vi "Totalize.vi"(6 "gain":dbl=1.0 format="%_6g", 7 "timebase":T1 items=["Seconds", "Minutes", "Hours", "Days"], 8 "error in":errorcluster, 9 "reset":bool, 10 "input":dbl format="%_6g", 11 "enable":bool=TRUE) -> (0 "error out":errorcluster, 3 "total":dbl format="%_6g")   [LabVIEW 2017, in "NI_FunctionBlock Libraries.lvlib"]
uses:
  <vilib>/functionblocks/NI_FunctionBlock Libraries.lvlib
  <vilib>/functionblocks/Accumulate/Totalize/Totalize.ctl
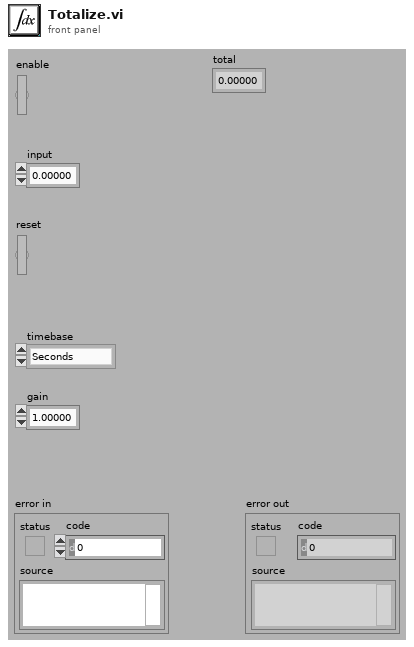
[diagram p1: front panel]
types:
  T1 = typedef "NI_FunctionBlock Libraries.lvlib/Totalize.ctl" = u16
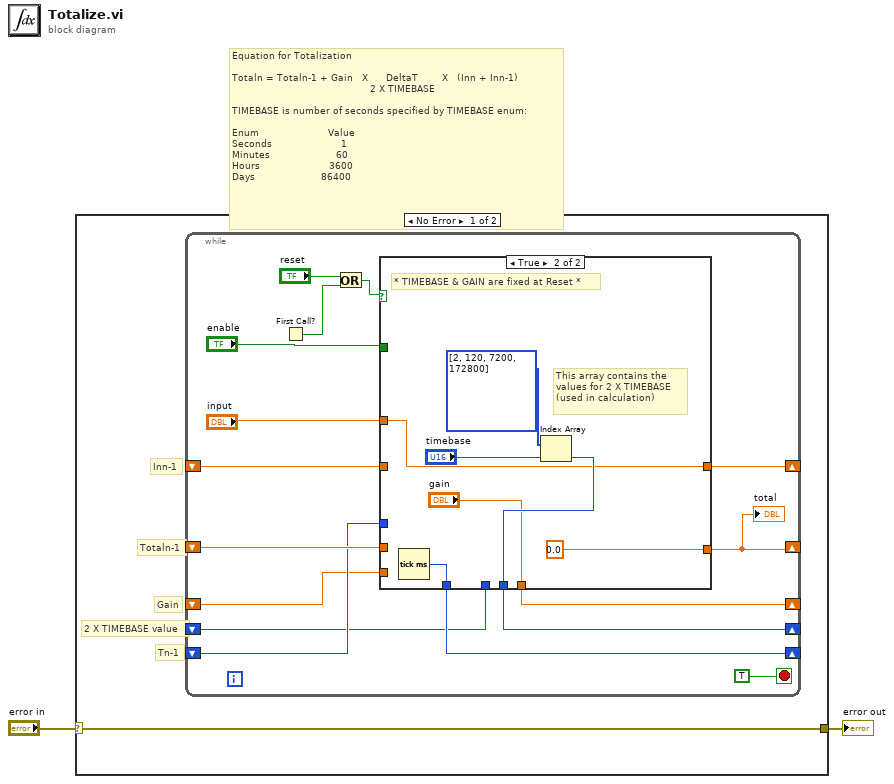
[diagram p0: block diagram]
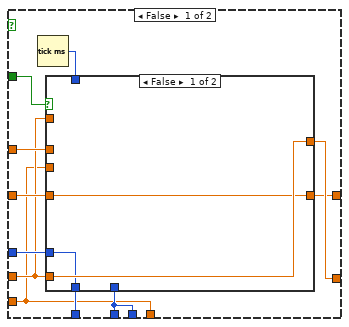
[diagram p2: hidden frame]
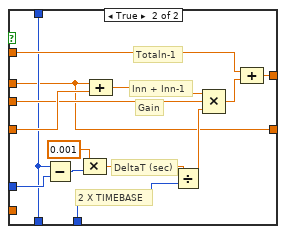
[diagram p3: hidden frame]
diagram:
  # "Equation for Totalization\n\nTotaln = Totaln-1 + Gain   X      DeltaT        X   (Inn + Inn-1)\n                                              2 X TIMEBASE\n\nTIMEBASE is number of seconds specified by TIMEBASE enum:\n\nEnum                       Value\nSeconds                       1\nMinutes                      60\nHours                       3600\nDays                      86400"
  n1 = case shown="No Error" "error in" {
    selector: "error in" -> [w3 w55]
    tunnel: [w3 w55] -> w1
    frame No Error {
      # "Gain"
      # "Tn-1"
      # "2 X TIMEBASE value"
      # "Totaln-1"
      # "Inn-1"
      n2 = while {
        shift-right: [w15] -> _
        shift-left: _ -> [w14]
        shift-right: [w4] -> _
        shift-left: _ -> [w13]
        shift-right: [w11] -> _
        shift-left: _ -> [w9]
        shift-right: [w10] -> _
        shift-left: _ -> [w12]
        shift-right: [w8] -> _
        shift-left: _ -> [w7]
        stop <- TRUE stop-if-true
        n3 = First Call?() -> (First Call?: T/F=w18:bool)
        n4 = Or(x="reset", y=w18) -> (x .or. y?=w17:bool)
        n5 = case shown="True" w17 {
          tunnel: [w28 0.0 ("Accumulation")] -> w15
          tunnel: "enable" -> [w30 _]
          tunnel: "input" -> [w29 w48]
          tunnel: w14 -> [w24 _]
          tunnel: w13 -> [w27 _]
          tunnel: w12 -> [w26 _]
          tunnel: [w23 w51] -> w11
          tunnel: [w25 w52] -> w10
          tunnel: w9 -> [w23 _]
          tunnel: [w21 "gain"] -> w8
          tunnel: w7 -> [w21 _]
          tunnel: [w20 w48] -> w4
          frame False {
            n6 = Tick Count (ms)() -> (millisecond timer value=w22:u32)
            n7 = case shown="False" w30 {
              tunnel: w29 -> [_ w34]
              tunnel: w24 -> [w33 _]
              tunnel: [w33 w41] -> w28
              tunnel: w27 -> [w32 w47]
              tunnel: w26 -> [w31 w45]
              tunnel: [w31 w37] -> w25
              tunnel: w23 -> [_ w38]
              tunnel: w21 -> [_ w43]
              tunnel: w24 -> [_ w39]
              tunnel: w22 -> [_ w37]
              tunnel: [w32 w34] -> w20
              frame False {
              }
              frame True {
                # "Totaln-1"
                # "Gain"
                # "Inn + Inn-1"
                # "2 X TIMEBASE"
                # "DeltaT (sec)"
                n8 = Subtract(x=w37, y=w45) -> (x-y=w44:u32)
                n9 = Compound Arithmetic op=MULTIPLY(0.001 ("value"), w44) -> (w36:dbl)
                n10 = Compound Arithmetic op=ADD(w34, w47) -> (w46:dbl)
                n11 = Divide(x=w36, y=w38) -> (x/y=w42:dbl)
                n12 = Compound Arithmetic op=MULTIPLY(w46, w43, w42) -> (w40:dbl)
                n13 = Compound Arithmetic op=ADD(w39, w40) -> (w41:dbl)
              }
            }
          }
          frame True {
            # "This array contains the\nvalues for 2 X TIMEBASE \n(used in calculation)"
            # "* TIMEBASE & GAIN are fixed at Reset *"
            n14 = Tick Count (ms)() -> (millisecond timer value=w52:u32)
            n15 = Index Array(array=u32[] [2, 120, 7200, 172800], index="timebase") -> (element=w51:u32)
          }
        }
        "total" <- w15
      }
    }
    frame Error {
    }
  }
  "error out" <- w1
